vi "svx_Orbit Legend Visible.vi"(6 "Bounds":T1, 7 "Bounds In":T2, 8 "Previous Visible?":bool, 9 "Legend Visible":bool, 10 "Legend Width":u32, 11 "Container":refnum<vi>) -> (5 "Bounds Out":cluster{"Width":u32, u32})   [LabVIEW 2017, in "SVX Orbit.xctl"]
uses:
  <vilib>/addons/_XControls/Orbit Plot/SVX Orbit.xctl
  <vilib>/addons/_XControls/Orbit Plot/subVIs/svx_Orbit Bounds.ctl
  <vilib>/Utility/miscctls.llb/LVBoundsTypeDef.ctl
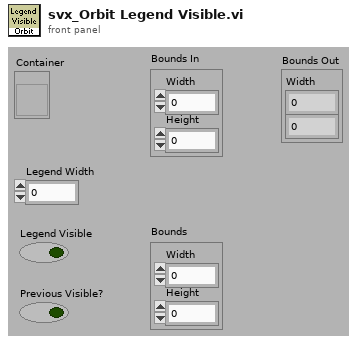
[diagram p1: front panel]
types:
  T1 = typedef "LVBoundsTypeDef.ctl" = cluster{"Width":u32, "Height":u32}
  T2 = typedef "SVX Orbit.xctl/svx_Orbit Bounds.ctl" = cluster{"Width":u32, "Height":u32}
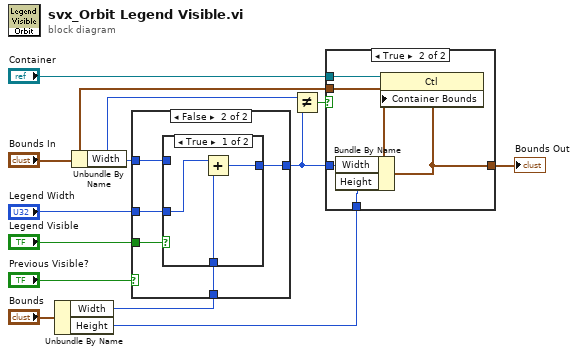
[diagram p0: block diagram]
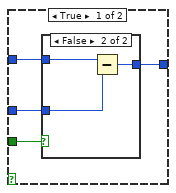
[diagram p3: hidden frame]
diagram:
  n1 = Unbundle By Name("Bounds") -> ("Width"=w1:u32, "Height"=w2:u32)
  n2 = Unbundle By Name("Bounds In") -> ("Width"=w6:u32)
  n3 = case shown="False" "Previous Visible?" {
    tunnel: "Legend Visible" -> [w16 w25]
    tunnel: "Legend Width" -> [w15 w22]
    tunnel: [w14 w24] -> w8
    tunnel: w6 -> [w13 w23]
    tunnel: w1 -> [_ w21]
    frame True {
      n4 = case shown="False" w16 {
        tunnel: w13 -> [w17 w20]
        tunnel: w15 -> [_ w19]
        tunnel: [w17 w18] -> w14
        frame True {
        }
        frame False {
          n5 = Subtract(x=w20, y=w19) -> (x-y=w18:u32)
        }
      }
    }
    frame False {
      n6 = case shown="True" w25 {
        tunnel: w23 -> [_ w29]
        tunnel: w22 -> [w27 _]
        tunnel: [w28 w29] -> w24
        tunnel: w21 -> [w26 _]
        frame True {
          n7 = Add(x=w27, y=w26) -> (x+y=w28:u32)
        }
        frame False {
        }
      }
    }
  }
  n8 = Not Equal?(x=w6, y=w8) -> (x != y?=w7:bool)
  n9 = case shown="True" w7 {
    tunnel: "Bounds In" -> [w30 w35]
    tunnel: "Container" -> [_ w34]
    tunnel: [w30 w33] -> w9
    tunnel: w8 -> [_ w32]
    tunnel: w2 -> [_ w31]
    frame False {
    }
    frame True {
      n10 = Bundle By Name(cluster=w35, "Width"=w32, "Height"=w31) -> (w33:T2)
      n11 = property class="Ctl"(reference=w34, "Container Bounds"=w33) -> ()  [unwired: 1 in, 2 out]
    }
  }
  "Bounds Out" <- w9
